vi "LabVIEWTempLogger.vi"() -> ()   [LabVIEW 2012]
uses:
  Instance           2 25Saved   LabVIEWTempLogger .vi
  Instance           1 25Saved   LabVIEWTempLogger .vi
  Instance           4 25Saved   LabVIEWTempLogger .vi
  Instance           3 25Saved   LabVIEWTempLogger .vi
panel:
  in  "Log Data?":bool=TRUE
  in  "Sampling Interval (s)":dbl=1.0 caption="Delay Time (s)"
  in  "File Path":path=path "C:/Users/Public/Documents/log.lvm" caption="Filename"
  out "Current Reading":dbl format="%#.1g"
  in  "Description":string="Enter a description"
  in  "Stop":bool
  out "Waveform Chart":dynamicdata(graph)=[{"t0"=timestamp(3371127248.414452 s since 1904-01-01), "dt"=1.0, "Y"=[23.308812327800272]}]
  # "NI USB-TC01 LabVIEW Temperature Logger"
  # "Switch to the block diagram (Window » Show Block Diagram) to configure the device, thermocouple type, and temperature unit."
  # "© 2010 National Instruments. All rights reserved."
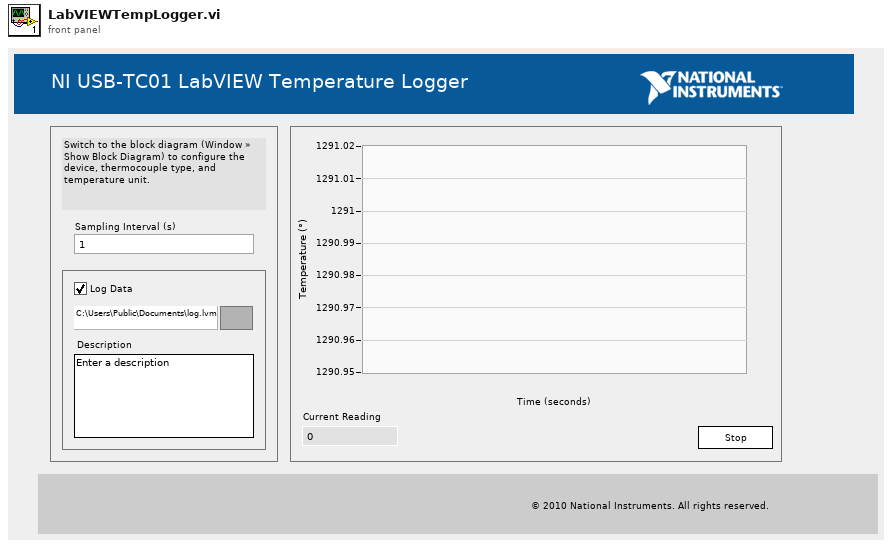
[diagram p1: front panel]
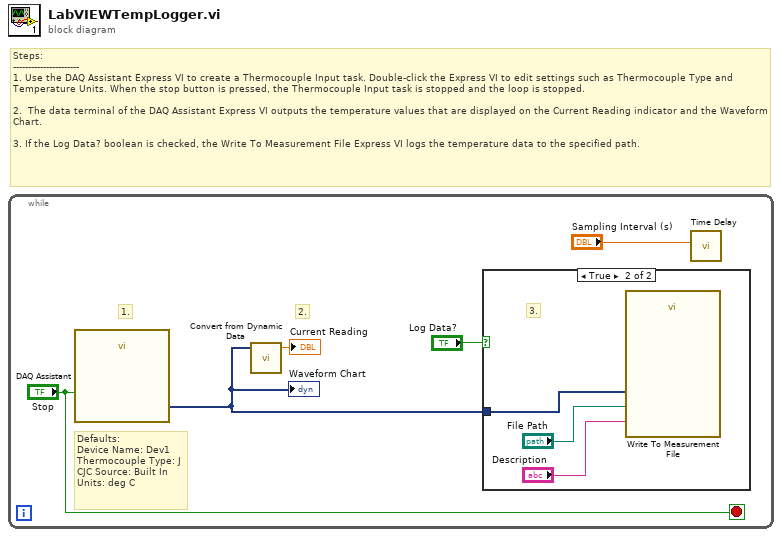
[diagram p0: block diagram]
diagram:
  # "Steps:\n----------------------\n1. Use the DAQ Assistant Express VI to create a Thermocouple Input task. Double-click the Express VI to edit settings such as Thermocouple Type and Temperature Units. When the stop button is pressed, the Thermocouple Input task is stopped and the loop is stopped.\n\n2.  The data terminal of the DAQ Assistant Express VI outputs the temperature values that are displayed on the Current Reading indicator and the Waveform Chart.\n\n3. If the Log Data? boolean is checked, the Write To Measurement File Express VI logs the temperature data to the specified path."
  n1 = while {
    stop <- "Stop" stop-if-true
    # "Defaults:\nDevice Name: Dev1\nThermocouple Type: J\nCJC Source: Built In\nUnits: deg C"
    # "2."
    # "1."
    n2 = call "DAQ Assistant"("stop (T)"="Stop") -> ("data"=w4:dynamicdata)  [unwired: 16 in, 2 out]
    "Waveform Chart" <- w4
    n3 = call "Convert from Dynamic Data"("Dynamic Data Type"=w4) -> ("Scalar"=→"Current Reading":dbl)  [unwired: 3 in]
    n4 = case shown="True" "Log Data?" {
      tunnel: w4 -> [_ w8]
      frame False {
      }
      frame True {
        # "3."
        n5 = call "Write To Measurement File"("Signals"=w8, "Filename"="File Path", "Comment"="Description") -> ()  [unwired: 14 in, 3 out]
      }
    }
    n6 = call "Time Delay"("Delay Time (s)"="Sampling Interval (s)") -> ()  [unwired: 10 in, 1 out]
  }
